vi "Set Pin.vi"(11 "Command to Send":string="SRC012;") -> (1 "Puerto":string, 2 "Pin":string, 3 "Valor pin":string)   [LabVIEW 2020, in "Test simulado.lvclass"]
uses:
  Test simulado.lvclass
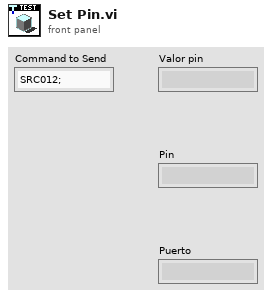
[diagram p1: front panel]
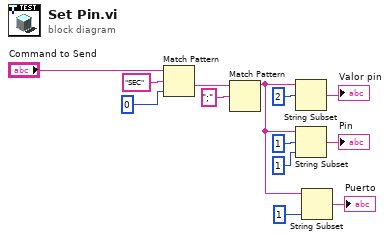
[diagram p0: block diagram]
diagram:
  n1 = Match Pattern(string="Command to Send", regular expression="SEC" ("string"), offset (0)=0) -> (after substring=w4:string)  [unwired: 3 out]
  n2 = Match Pattern(string=w4, regular expression=";") -> (before substring=w9:string)  [unwired: 1 in, 3 out]
  n3 = String Subset(string=w9, offset (0)=2) -> (substring=→"Valor pin":string)  [unwired: 1 in]
  n4 = String Subset(string=w9, offset (0)=1, length (rest)=1 ("length (rest)")) -> (substring=→"Pin":string)
  n5 = String Subset(string=w9, length (rest)=1 ("length (rest)")) -> (substring=→"Puerto":string)  [unwired: 1 in]
